vi "Waveform Time Ramp.vi"(8 "Error In":errorcluster, 10 "End [s]":dbl, 11 "dt [s]":dbl) -> (0 "Error Out":errorcluster, 1 "Waveform Time Ramp":waveform(dbl))   [LabVIEW 2021]
uses:
  <vilib>/Analysis/1siggen.llb/Ramp Pattern by Delta.vi
  <vilib>/Analysis/NI_AALBase.lvlib
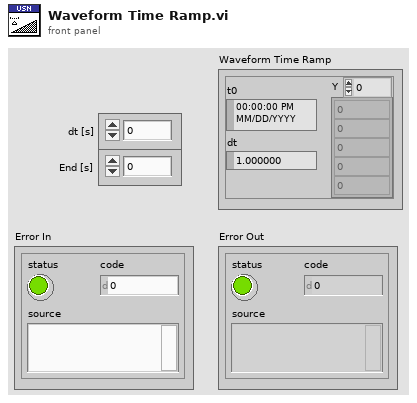
[diagram p1: front panel]
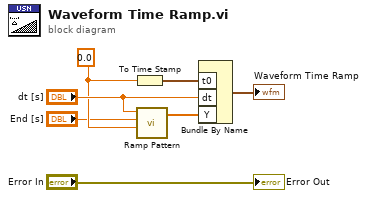
[diagram p0: block diagram]
diagram:
  w5 = 0.0 ("start")
  n1 = To Time Stamp(1:w5) -> (0:w3:timestamp)
  n2 = call-poly <vilib>:"Ramp Pattern.vi"("start"=w5, "end"="End [s]", "delta"="dt [s]") -> ("Ramp Pattern"=w7:dbl[])  [unwired: 6 in, 2 out]
  n3 = Bundle By Name("t0"=w3, "dt"="dt [s]", "Y"=w7) -> (→"Waveform Time Ramp":waveform(dbl))  [unwired: 1 in]
  "Error Out" <- "Error In"
